vi "tic tac toe VI group.vi"() -> ()   [LabVIEW 2019]
uses:
  typedefs/tic-tac-toe board.ctl
  typedefs/x or o or empty.ctl
  typedefs/invisible buttons.ctl
  typedefs/game status.ctl
  typedefs/turn enum.ctl
  typedefs/tic-tac-toe state enum.ctl
  typedefs/tic-tac-toe data.ctl
panel:
  out "desired move":bool[][](array[boolean])=[[FALSE, FALSE, FALSE], [FALSE, TRUE, FALSE], [FALSE, FALSE, FALSE]]
  out "eval board":i32[][](array[numeric])=[[0, 1, -1], [0, 0, 0], [0, 0, 0]]
  out "display board":u16[][](array[numeric])=[[0, 1, 2], [0, 0, 0], [0, 0, 0]]
  in  "tic tac toe data":T1={"state"=enum."start game", "display board"=[[0, 1, 2], [0, 0, 0], [0, 0, 0]], "eval board"=[[0, 1, -1], [0, 0, 0], [0, 0, 0]], "turn"=enum."x turn", "desired move"=[[FALSE, FALSE, FALSE], [FALSE, TRUE, FALSE], [FALSE, FALSE, FALSE]], "game status"=enum."not over"}
  out "state":T2
  out "turn":T3
  out "game status":T4
  in  "invisible buttons":T5
  out "pict ring":T6=1 caption="Ring"
  out "game board":T7=[[0, 1, 2], [0, 0, 0], [0, 0, 0]]
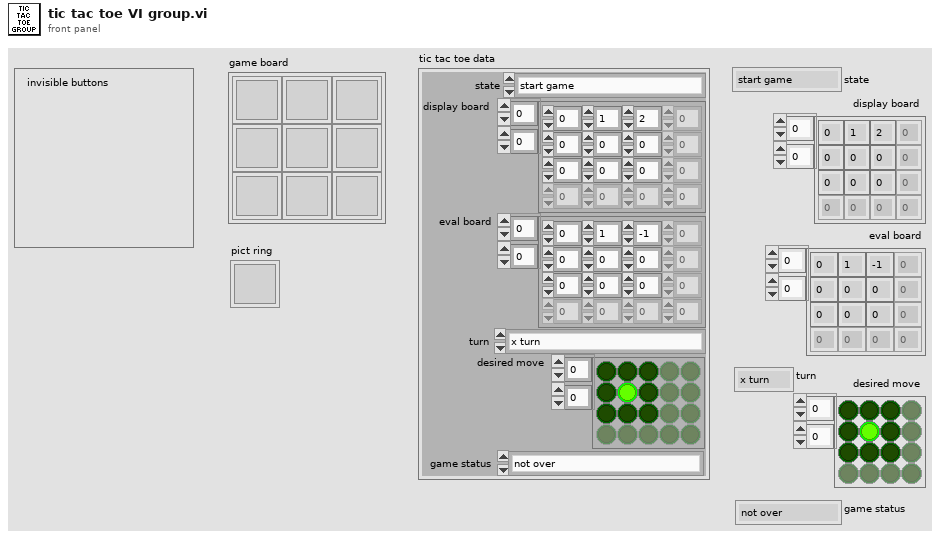
[diagram p1: front panel]
types:
  T1 = typedef "tic-tac-toe data.ctl" = cluster{"state":T2, "display board":u16[][], "eval board":i32[][], "turn":T3, "desired move":bool[][], "game status":T4}
  T2 = typedef "tic-tac-toe state enum.ctl" = enum16{"start game", "clear", "x turn", "o turn", "legal move", "update board", "evaluate board", "turn decide", "game over"}
  T3 = typedef "turn enum.ctl" = enum32{"x turn", "o turn"}
  T4 = typedef "game status.ctl" = enum16{"not over", "over stalemate", "over x wins", "over o wins"}
  T5 = typedef "invisible buttons.ctl" = cluster{"00":bool, "01":bool, "02":bool, "10":bool, "11":bool, "12":bool, "20":bool, "21":bool, "22":bool}
  T6 = typedef "x or o or empty.ctl" = u16
  T7 = typedef "tic-tac-toe board.ctl" = T6[][]
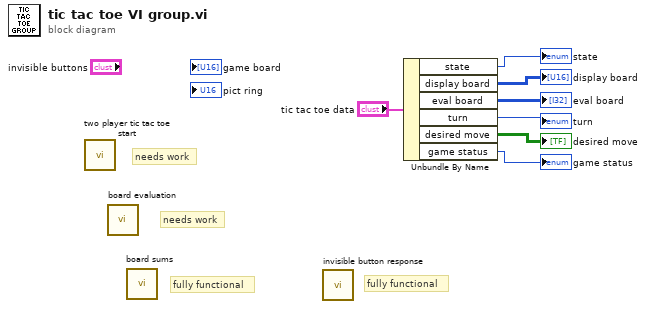
[diagram p0: block diagram]
diagram:
  # "fully functional"
  # "needs work"
  # "fully functional"
  # "needs work"
  n1 = call "two player tic tac toe start.vi"() -> ()  [unwired: 1 in]
  n2 = call "board evaluation.vi"() -> ()  [unwired: 15 in, 1 out]
  n3 = call "board sums.vi"() -> ()  [unwired: 15 in, 1 out]
  n4 = call "invisible button response.vi"() -> ()  [unwired: 14 in, 2 out]
  n5 = Unbundle By Name("tic tac toe data") -> ("state"=→"state":T2, "display board"=→"display board":u16[][], "eval board"=→"eval board":i32[][], "turn"=→"turn":T3, "desired move"=→"desired move":bool[][], "game status"=→"game status":T4)
